vi "Numeric Controls and Indicators.vi"() -> ()   [LabVIEW 2010]
doc: "This is a sample VI used to demonstrate basic functions on the LabVIEW block diagram."
panel:
  out "Indicator":dbl
  in  "Control 2":dbl min=0.0 max=100.0 step=1.0
  in  "Control 1":dbl
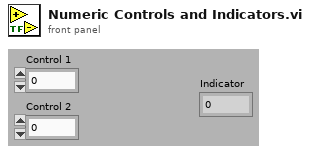
[diagram p1: front panel]
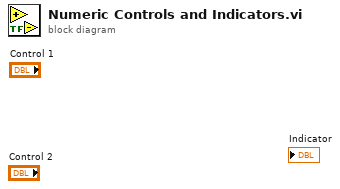
[diagram p0: block diagram]
diagram:
